vi "TEST Object Manual Bounds (Advanced Interactive Splitter).vi"() -> ()   [LabVIEW 2021, in "IObject.lvclass"]
uses:
  IObject.lvclass
  IContainer/Divider/Divider.lvclass
  C:/Projects/Dynamic-Scaling/Dynamic Scaling/IObject.lvclass
  Object/Object.lvclass
  IContainer/Viewport/Viewport.lvclass
  C:/Projects/Dynamic-Scaling/Dynamic Scaling/IContainer/IContainer.lvclass
  IContainer/Divider/Splitter/Splitter.lvclass
  C:/Projects/Dynamic-Scaling/Dynamic Scaling/IContainer/Divider/Divider.lvclass
  IContainer/IContainer.lvclass
  IContainer/Interaction/Interaction.lvclass
panel:
  out "In Object":string[](array[string])
  out "Status":string
  out "Resized":string[](array[string])
  out "XY Graph 6":cluster{"X":dbl, "Y":dbl}[](graph)
  out "XY Graph 5":cluster{"X":dbl, "Y":dbl}[](graph)
  out "XY Graph 4":cluster{"X":dbl, "Y":dbl}[](graph)
  out "XY Graph 3":cluster{"X":dbl, "Y":dbl}[](graph)
  out "XY Graph 2":cluster{"X":dbl, "Y":dbl}[](graph)
  out "XY Graph":cluster{"X":dbl, "Y":dbl}[](graph)
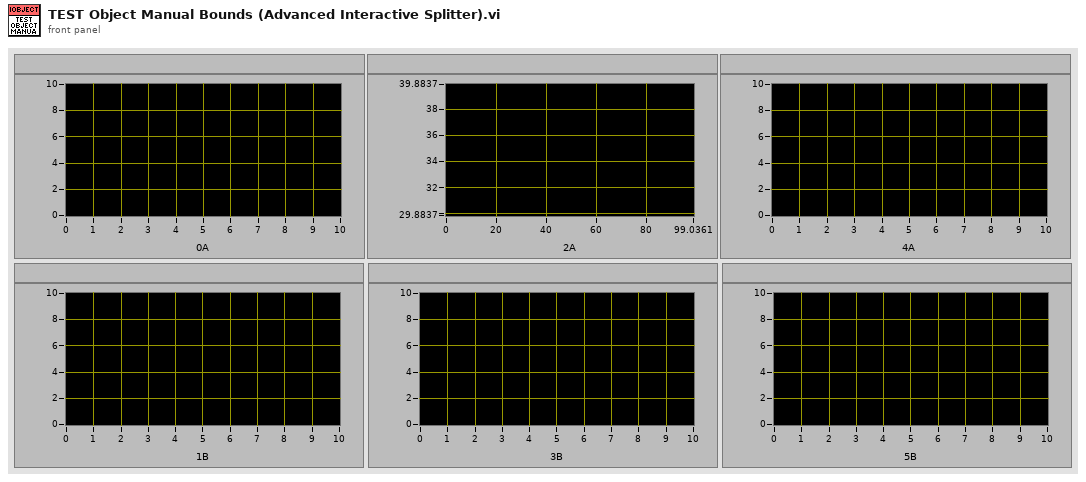
[diagram p1: front panel]
types:
  T1 = cluster{"Left":dbl, "Top":dbl, "Right":dbl, "Bottom":dbl}
  T2 = typedef "LVRectTypeDef.ctl" = cluster{"Left":i16, "Top":i16, "Right":i16, "Bottom":i16}
  T3 = typedef "LVPoint32TypeDef.ctl" = cluster{"Horizontal":i32, "Vertical":i32}
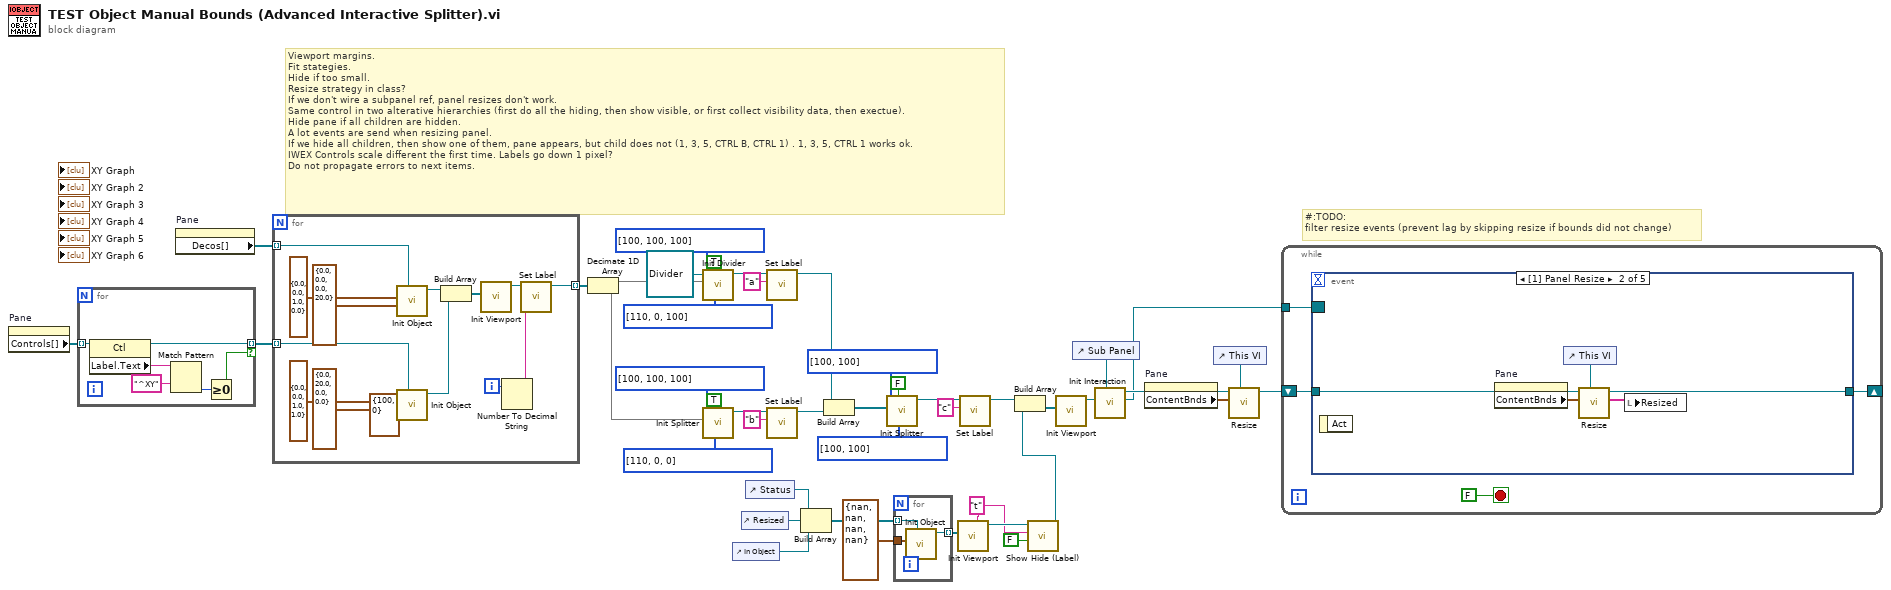
[diagram p0: block diagram]
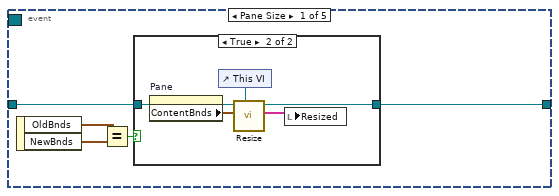
[diagram p2: hidden frame]
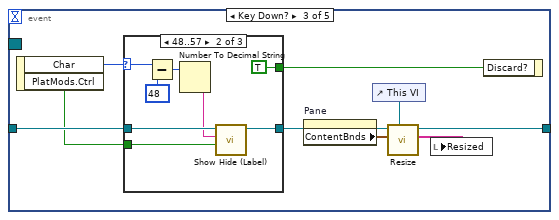
[diagram p4: hidden frame]
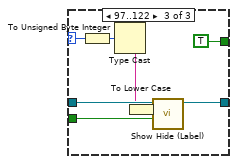
[diagram p6: hidden frame]
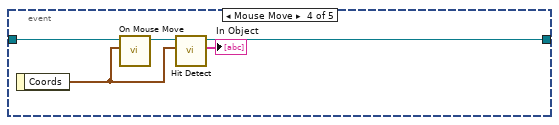
[diagram p7: hidden frame]
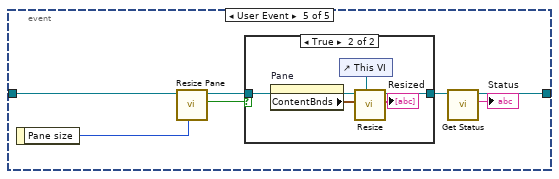
[diagram p8: hidden frame]
diagram:
  w2 = "t" ("Label")
  # "#:TODO:\nfilter resize events (prevent lag by skipping resize if bounds did not change)"
  # "Viewport margins.\nFit stategies.\nHide if too small.\nResize strategy in class?\nIf we don't wire a subpanel ref, panel resizes don't work.\nSame control in two alterative hierarchies (first do all the hiding, then show visible, or first collect visibility data, then exectue).\nHide pane if all children are hidden.\nA lot events are send when resizing panel.\nIf we hide all children, then show one of them, pane appears, but child does not (1, 3, 5, CTRL B, CTRL 1) . 1, 3, 5, CTRL 1 works ok.\nIWEX Controls scale different the first time. Labels go down 1 pixel?\nDo not propagate errors to next items."
  n1 = property on="Pane" class="Pane"() -> ("Controls[]"=w22:refnum<vi>[])  [unwired: 2 in, 2 out]
  n2 = for {
    tunnel: w22 -> [w50] mode=indexing
    tunnel: [w47] -> w21 mode=indexing if=w45
    n3 = property class="Ctl"(reference=w50) -> (reference out=w47:refnum<vi>, "Label.Text"=w49:string)  [unwired: 1 in, 1 out]
    n4 = Match Pattern(string=w49, regular expression="^XY") -> (offset past match=w46:i32)  [unwired: 1 in, 3 out]
    n5 = Greater Or Equal To 0?(x=w46) -> (x >= 0?=w45:bool)
  }
  n6 = property on="Pane" class="Pane"() -> ("Decos[]"=w42:refnum<vi>[])  [unwired: 2 in, 2 out]
  n7 = for {
    tunnel: w42 -> [w64] mode=indexing
    tunnel: [w53] -> w37 mode=indexing
    tunnel: w21 -> [w57] mode=indexing
    i -> [w63]
    n8 = call "Init Object.vi"("GObj Refnum"=w64, "B [0, 0, 0, 0]"=T1 {"Left"=0.0, "Top"=0.0, "Right"=0.0, "Bottom"=20.0} ("B"), "A [0, 0, 1, 1]"=T1 {"Left"=0.0, "Top"=0.0, "Right"=1.0, "Bottom"=0.0} ("A")) -> ("MMI Scaling out"=w55:refnum<class "Object.lvclass">)  [unwired: 7 in, 1 out]
    n9 = call "Init Object.vi"("Minimal size [0, 0]"=cluster{"Horizontal":i16, "Vertical":i16} {"Horizontal"=100, "Vertical"=0}, "GObj Refnum"=w57, "B [0, 0, 0, 0]"=T1 {"Left"=0.0, "Top"=20.0, "Right"=0.0, "Bottom"=0.0} ("B"), "A [0, 0, 1, 1]"=T1 {"Left"=0.0, "Top"=0.0, "Right"=1.0, "Bottom"=1.0} ("A")) -> ("MMI Scaling out"=w54:refnum<class "Object.lvclass">)  [unwired: 6 in, 1 out]
    n10 = Build Array(w55, w54) -> (w60:refnum<class "Object.lvclass">[])
    n11 = call "Init Viewport.vi"("Items"=w60) -> ("Viewport out"=w52:refnum<class "Viewport.lvclass">)  [unwired: 9 in, 1 out]
    n12 = Number To Decimal String(number=w63) -> (decimal integer string=w56:string)  [unwired: 1 in]
    n13 = call "Set Label.vi"("Label"=w56, "MMI Scaling in"=w52) -> ("MMI Scaling out"=w53:refnum<class "Viewport.lvclass">)  [unwired: 8 in, 1 out]
  }
  n14 = Decimate 1D Array(w37) -> (w38:refnum<class "Viewport.lvclass">[], w31:refnum<class "Viewport.lvclass">[])
  n15 = call "Init Divider.vi"("Minimal size"=i16[] [110, 0, 100], "Vertical? [F, hor.]"=TRUE, "Relative size"=i16[] [100, 100, 100] ("Minimal size"), "Items"=w38, "Divider in"=refnum<class "Divider.lvclass"> refnum) -> ("Divider out"=w44:refnum<class "Divider.lvclass">)  [unwired: 5 in, 1 out]
  n16 = call "Init Splitter.vi"("Minimal size"=i16[] [110, 0, 0], "Vertical? [F, hor.]"=TRUE, "Relative size"=i16[] [100, 100, 100] ("Minimal size"), "Items"=w31) -> ("Splitter out"=w32:refnum<class "Splitter.lvclass">)  [unwired: 6 in, 1 out]
  n17 = control-ref of="In Object"() -> (w7:refnum<vi>)
  n18 = control-ref of="Resized"() -> (w8:refnum<vi>)
  n19 = control-ref of="Status"() -> (w9:refnum<vi>)
  n20 = call "Set Label.vi"("Label"="a", "MMI Scaling in"=w44) -> ("MMI Scaling out"=w28:refnum<class "Divider.lvclass">)  [unwired: 8 in, 1 out]
  n21 = call "Set Label.vi"("Label"="b", "MMI Scaling in"=w32) -> ("MMI Scaling out"=w30:refnum<class "Splitter.lvclass">)  [unwired: 8 in, 1 out]
  n22 = Build Array(w9, w8, w7) -> (w5:refnum<vi>[])
  n23 = Build Array(w28, w30) -> (w29:refnum<class "Divider.lvclass">[])
  n24 = call "Init Splitter.vi"("Minimal size"=i16[] [100, 100] ("Size"), "Vertical? [F, hor.]"=FALSE, "Relative size"=i16[] [100, 100] ("Size"), "Items"=w29) -> ("Splitter out"=w23:refnum<class "Splitter.lvclass">)  [unwired: 6 in, 1 out]
  n25 = for {
    tunnel: T1 {"Left"=nan, "Top"=nan, "Right"=nan, "Bottom"=nan} ("A [0, 0, 1, 1]") -> [w67]
    tunnel: [w66] -> w6 mode=indexing
    tunnel: w5 -> [w65] mode=indexing
    n26 = call "Init Object.vi"("GObj Refnum"=w65, "A [0, 0, 1, 1]"=w67) -> ("MMI Scaling out"=w66:refnum<class "Object.lvclass">)  [unwired: 8 in, 1 out]
  }
  n27 = call "Init Viewport.vi"("Label"=w2, "Items"=w6) -> ("Viewport out"=w4:refnum<class "Viewport.lvclass">)  [unwired: 8 in, 1 out]
  n28 = call "Set Label.vi"("Label"="c", "MMI Scaling in"=w23) -> ("MMI Scaling out"=w12:refnum<class "Splitter.lvclass">)  [unwired: 8 in, 1 out]
  n29 = call-dynamic "Show Hide (Label).vi"("Show? [T]"=FALSE, "Label"=w2, "MMI Scaling in"=w4) -> ("MMI Scaling out"=w3:refnum<class "Viewport.lvclass">)  [unwired: 6 in, 2 out]
  n30 = Build Array(w12, w3) -> (w11:refnum<class "IContainer.lvclass">[])
  n31 = call "Init Viewport.vi"("Items"=w11) -> ("Viewport out"=w13:refnum<class "Viewport.lvclass">)  [unwired: 9 in, 1 out]
  n32 = control-ref of="Sub Panel"() -> (w20:refnum<vi>)
  n33 = call "Init Interaction.vi"("Sub Panel"=w20, "IObject"=w13) -> ("Interaction Splitter Resize"=w15:refnum<event-registration>, "Interaction out"=w17:refnum<class "Interaction.lvclass">)  [unwired: 6 in, 2 out]
  n34 = property on="Pane" class="Pane"() -> ("ContentBnds"=w18:T2)  [unwired: 2 in, 2 out]
  n35 = control-ref of="This VI"() -> (w19:refnum<vi>)
  n36 = call-dynamic "Resize.vi"("VI Refnum"=w19, "Bounds"=w18, "MMI Scaling in"=w17) -> ("MMI Scaling out"=w16:refnum<class "Interaction.lvclass">)  [unwired: 6 in, 2 out]
  n37 = while {
    shift-right: [w69] -> _
    shift-left: w16 -> [w71]
    tunnel: w15 -> [w68]
    stop <- FALSE stop-if-true
    n38 = event shown="[1] Panel Resize" {
      selector: w68 -> [_ _ _ _ _]
      dyn-events: _ -> [_ _ _ _ _]
      timeout: _ -> [_ _ _ _ _]
      tunnel: w71 -> [w76 w87 w92 w118 w125]
      tunnel: [w75 w86 w89 w116 w120] -> w69
      event Pane Size {
        n39 = event-data() -> ("OldBnds"=w74:T2, "NewBnds"=w73:T2)  [unwired: 1 in]
        n40 = Equal?(x=w74, y=w73) -> (x = y?=w72:bool)
        n41 = case shown="True" w72 {
          tunnel: w76 -> [w77 w82]
          tunnel: [w77 w79] -> w75
          frame False {
          }
          frame True {
            n42 = property on="Pane" class="Pane"() -> ("ContentBnds"=w81:T2)  [unwired: 2 in, 2 out]
            n43 = control-ref of="This VI"() -> (w80:refnum<vi>)
            n44 = call-dynamic "Resize.vi"("VI Refnum"=w80, "Bounds"=w81, "MMI Scaling in"=w82) -> ("Resized"=w78:string[], "MMI Scaling out"=w79:refnum<class "Interaction.lvclass">)  [unwired: 6 in, 1 out]
            n45 = local write "Resized"(w78) -> ()
          }
        }
      }
      event Panel Resize {
        n46 = event-data() -> ()  [unwired: 1 in, 1 out]
        n47 = property on="Pane" class="Pane"() -> ("ContentBnds"=w85:T2)  [unwired: 2 in, 2 out]
        n48 = control-ref of="This VI"() -> (w84:refnum<vi>)
        n49 = call-dynamic "Resize.vi"("VI Refnum"=w84, "Bounds"=w85, "MMI Scaling in"=w87) -> ("Resized"=w83:string[], "MMI Scaling out"=w86:refnum<class "Interaction.lvclass">)  [unwired: 6 in, 1 out]
        n50 = local write "Resized"(w83) -> ()
      }
      event Key Down? {
        n51 = event-data() -> ("Char"=w94:i16, "PlatMods.Ctrl"=w91:bool)  [unwired: 1 in]
        n52 = case shown="48..57" w94 {
          selector: w94 -> [_ w105 w111]
          tunnel: [w97 w101 w112] -> w93
          tunnel: w92 -> [w97 w103 w113]
          tunnel: w91 -> [_ w100 w109]
          tunnel: [_ TRUE TRUE] -> w88
          frame Default {
          }
          frame 48..57 {
            n53 = Subtract(x=w105, y=i16 48) -> (x-y=w102:i16)
            n54 = Number To Decimal String(number=w102) -> (decimal integer string=w99:string)  [unwired: 1 in]
            n55 = call-dynamic "Show Hide (Label).vi"("Show? [T]"=w100, "Label"=w99, "MMI Scaling in"=w103) -> ("MMI Scaling out"=w101:refnum<class "Interaction.lvclass">)  [unwired: 6 in, 2 out]
          }
          frame 97..122 {
            n56 = To Unsigned Byte Integer(number=w111) -> (unsigned 8bit integer=w110:u8)
            n57 = Type Cast(x=w110) -> (*(type *) &x=w108:string)  [unwired: 1 in]
            n58 = To Lower Case(string=w108) -> (all lower case string=w107:string)
            n59 = call-dynamic "Show Hide (Label).vi"("Show? [T]"=w109, "Label"=w107, "MMI Scaling in"=w113) -> ("MMI Scaling out"=w112:refnum<class "Interaction.lvclass">)  [unwired: 6 in, 2 out]
          }
        }
        n60 = property on="Pane" class="Pane"() -> ("ContentBnds"=w96:T2)  [unwired: 2 in, 2 out]
        n61 = control-ref of="This VI"() -> (w95:refnum<vi>)
        n62 = call-dynamic "Resize.vi"("VI Refnum"=w95, "Bounds"=w96, "MMI Scaling in"=w93) -> ("Resized"=w90:string[], "MMI Scaling out"=w89:refnum<class "Interaction.lvclass">)  [unwired: 6 in, 1 out]
        n63 = local write "Resized"(w90) -> ()
        n64 = event-data("Discard?"=w88) -> ()  [unwired: 1 in, 1 out]
      }
      event Mouse Move {
        n65 = event-data() -> ("Coords"=w115:T3)  [unwired: 1 in]
        n66 = call "On Mouse Move.vi"("Coords"=w115, "Interaction in"=w118) -> ("Interaction out"=w117:refnum<class "Interaction.lvclass">)  [unwired: 8 in, 1 out]
        n67 = call-dynamic "Hit Detect.vi"("Coords"=w115, "IContainer in"=w117) -> ("In Object"=→"In Object":string[], "IContainer out"=w116:refnum<class "Interaction.lvclass">)  [unwired: 6 in, 2 out]
      }
      event User Event {
        n68 = event-data() -> ("Pane size"=w124:i32)  [unwired: 1 in]
        n69 = call-dynamic "Resize Pane.vi"("Pane size"=w124, "IContainer in"=w125) -> ("Resized?"=w123:bool, "IContainer out"=w122:refnum<class "Interaction.lvclass">)  [unwired: 7 in, 1 out]
        n70 = case shown="True" w123 {
          tunnel: [w126 w129] -> w119
          tunnel: w122 -> [w126 w128]
          frame False {
          }
          frame True {
            n71 = property on="Pane" class="Pane"() -> ("ContentBnds"=w131:T2)  [unwired: 2 in, 2 out]
            n72 = control-ref of="This VI"() -> (w130:refnum<vi>)
            n73 = call-dynamic "Resize.vi"("VI Refnum"=w130, "Bounds"=w131, "MMI Scaling in"=w128) -> ("Resized"=→"Resized":string[], "MMI Scaling out"=w129:refnum<class "Interaction.lvclass">)  [unwired: 6 in, 1 out]
          }
        }
        n74 = call-dynamic "Get Status.vi"("IContainer in"=w119) -> ("Status"=→"Status":string, "IContainer out"=w120:refnum<class "Interaction.lvclass">)  [unwired: 8 in, 1 out]
      }
    }
  }
